vi "Task DAQ.vi"() -> ()   [LabVIEW 2025]
uses:
  <vilib>/DAQmx/write.llb/DAQmx Write (Digital Bool 1Line 1Point).vi
  <vilib>/DAQmx/read.llb/DAQmx Read (Digital Bool 1Line 1Point).vi
panel:
  in  "Stop":bool
  out "Read":bool
  in  "Write":bool
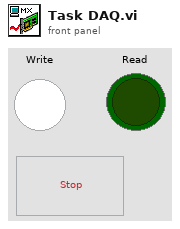
[diagram p1: front panel]
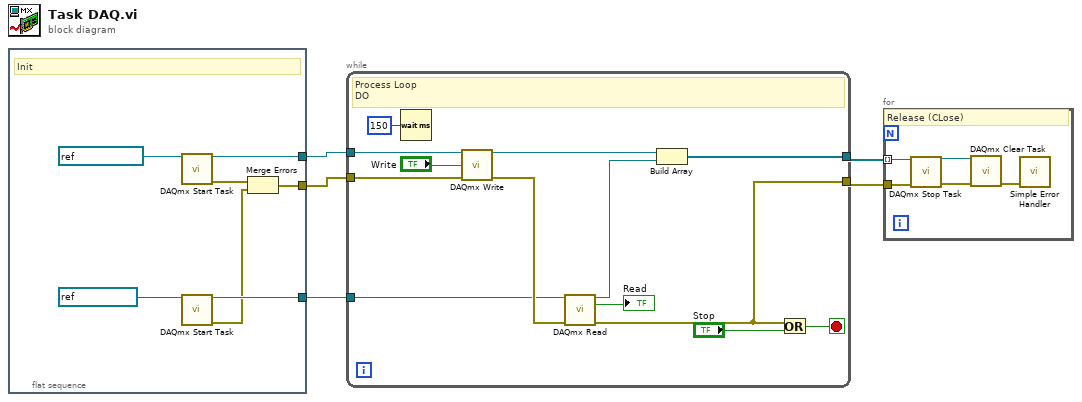
[diagram p0: block diagram]
diagram:
  n1 = flat-sequence {
    tunnel: [w11] -> w5
    tunnel: [w9] -> w2
    tunnel: [w7] -> w1
    frame #0 {
      # "Init"
      n2 = call <vilib>:"DAQmx Start Task.vi"("task/channels in"=refnum<k21> "DO 0 Cdaq" ("DAQmx Task Name")) -> ("task out"=w11:refnum<k21>, "error out"=w10:errorcluster)  [unwired: 13 in]
      n3 = call <vilib>:"DAQmx Start Task.vi"("task/channels in"=refnum<k21> "DI 1 Cdaq" ("DAQmx Task Name")) -> ("task out"=w9:refnum<k21>, "error out"=w6:errorcluster)  [unwired: 13 in]
      n4 = Merge Errors(w10, w6) -> (w7:errorcluster)
    }
  }
  n5 = while {
    tunnel: w5 -> [w25]
    tunnel: w1 -> [w23]
    tunnel: [w14] -> w4
    tunnel: [w17] -> w3
    tunnel: w2 -> [w16]
    stop <- w19 stop-if-true
    # "Process Loop\nDO"
    n6 = Wait (ms)(milliseconds to wait=u32 150) -> ()  [unwired: 1 out]
    n7 = call-poly <vilib>:"DAQmx Write.vi"("task/channels in"=w25, "data"="Write", "error in"=w23) -> ("task out"=w21:refnum<k21>, "error out"=w18:errorcluster)  [unwired: 10 in, 1 out]
    n8 = call-poly <vilib>:"DAQmx Read.vi"("task/channels in"=w16, "error in"=w18) -> ("task out"=w13:refnum<k21>, "data"=→"Read":bool, "error out"=w17:errorcluster)  [unwired: 11 in]
    n9 = Build Array(w21, w13) -> (w14:refnum<k21>[])
    n10 = Or(x=w17, y="Stop") -> (x .or. y?=w19:bool)
  }
  n11 = for {
    tunnel: w4 -> [w30] mode=indexing
    tunnel: w3 -> [w29]
    # "Release (CLose)"
    n12 = call <vilib>:"DAQmx Stop Task.vi"("task/channels in"=w30, "error in"=w29) -> ("task out"=w27:refnum<k21>, "error out"=w28:errorcluster)  [unwired: 12 in]
    n13 = call <vilib>:"DAQmx Clear Task.vi"("task in"=w27, "error in"=w28) -> ("error out"=w26:errorcluster)  [unwired: 13 in]
    n14 = call <vilib>:"Simple Error Handler.vi"("error in (no error)"=w26) -> ()  [unwired: 4 in, 5 out]
  }
